vi "read temp.vi"() -> ()   [LabVIEW 2016]
uses:
  <vilib>/Instr/_visa.llb/VISA Configure Serial Port (Instr).vi
panel:
  out "Temperature":dbl[][](graph)
  out "Heater Power":dbl[](graph)
  out "Heater Power":string
  in  "Heater Range":u16(ring) items=["Off", "Low", "Med", "High"]
  in  "Target Temperature":i32
  out "?":string
  out "bytes read":u32
  in  "Set Temperature and heater range":bool
  out "Actual Temperature":string
  in  "Stop Programme":bool
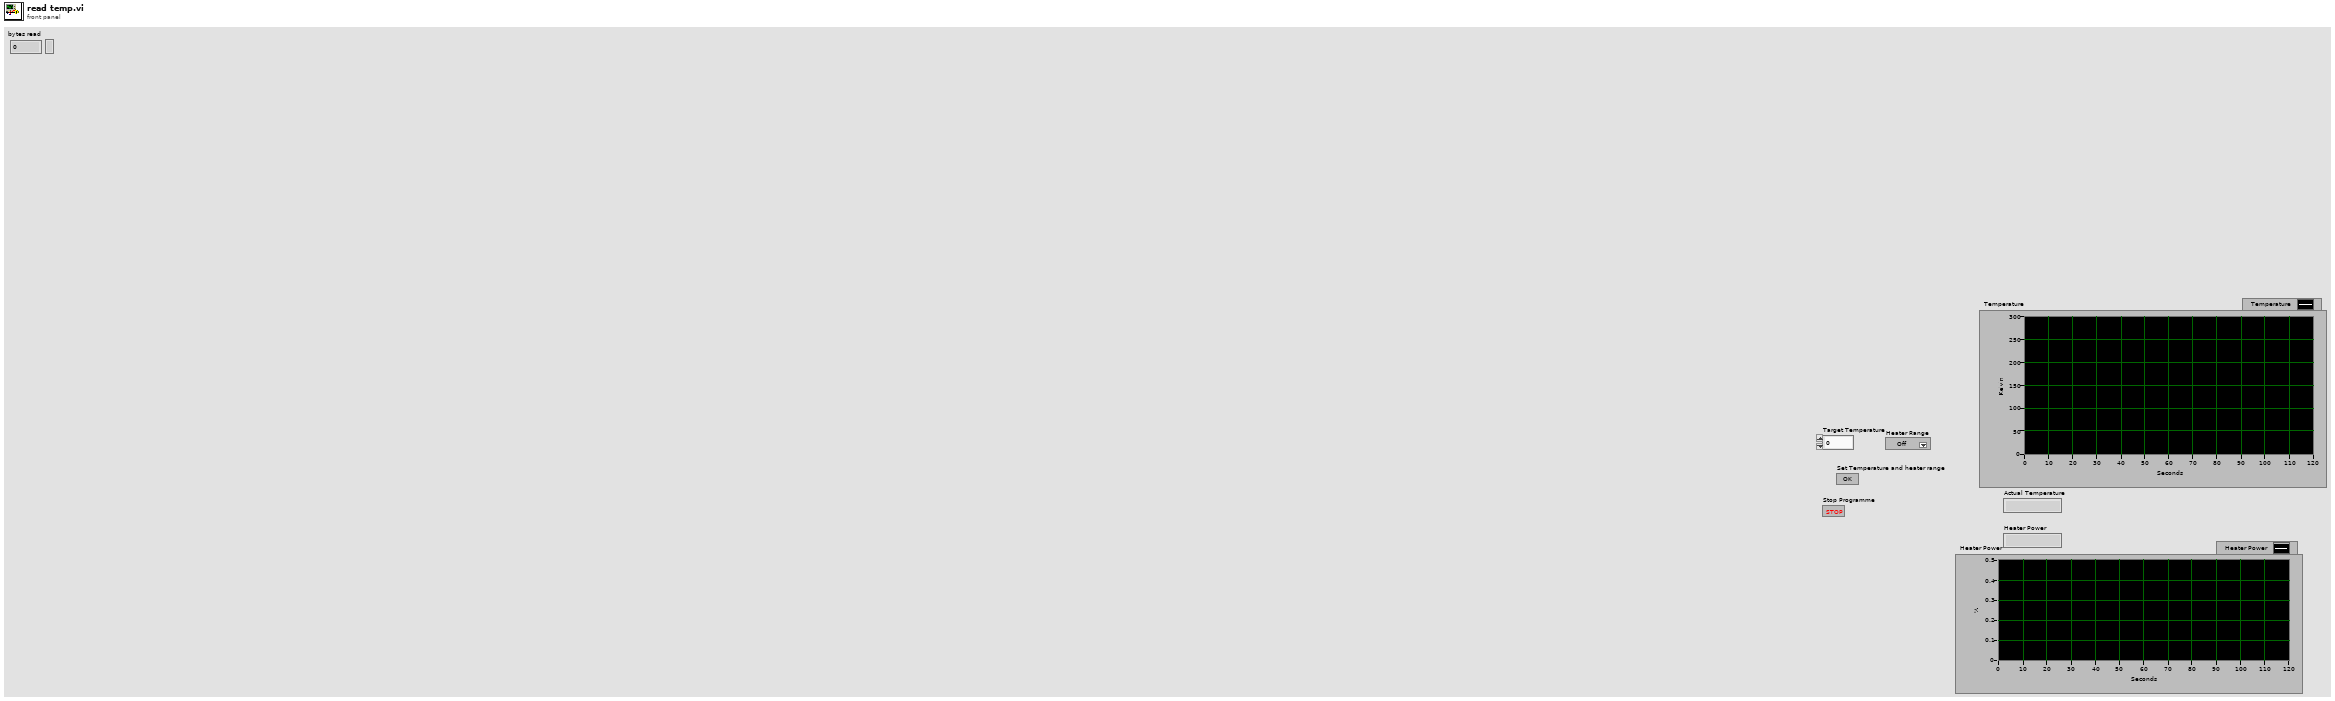
[diagram p1: front panel]
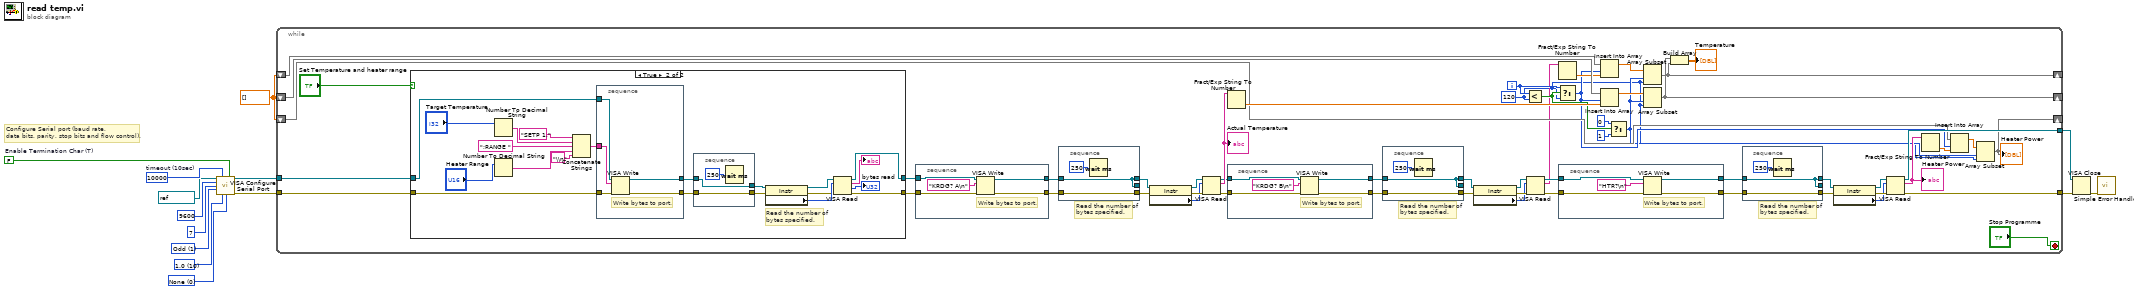
[diagram p0: block diagram]
diagram:
  w1 = dbl[] []
  w7 = u16 0 items=["None"=0, "XON/XOFF"=1, "RTS/CTS"=2, "DTR/DSR"=4] ("flow control")
  w8 = u16 10 items=["1.0"=10, "1.5"=15, "2.0"=20] ("stop bits")
  w9 = u16 1 items=["None", "Odd", "Even", "Mark", "Space"] ("parity")
  w13 = FALSE  # Enable Termination Char (T)
  w14 = u32 10000  # timeout (10sec)
  # "Configure Serial port (baud rate,\ndata bits, parity, stop bits and flow control)."
  n1 = call-poly "VISA Configure Serial Port"("VISA resource name"=refnum<visa-resource-name> "COM3", "timeout (10sec)"=w14, "Enable Termination\nChar (T)"=w13, "baud rate (9600)"=u32 9600 ("baud rate"), "data bits (8)"=u16 7 ("data bits"), "parity (0:none)"=w9, "stop bits (10: 1 bit)"=w8, "flow control (0:none)"=w7) -> ("VISA resource name out"=w5:refnum<visa-resource-name>, "error out"=w4:errorcluster)  [unwired: 1 in, 5 out]
  n2 = while {
    tunnel: w5 -> [w61]
    tunnel: w4 -> [w60]
    tunnel: [w42] -> w3
    tunnel: [w41] -> w2
    shift-right: [w17] -> _
    shift-left: w1 -> [w55]
    shift-right: [w37] -> _
    shift-left: w1 -> [w36]
    shift-right: [w16] -> _
    shift-left: w1 -> [w15]
    i -> [w53]
    stop <- "Stop Programme" stop-if-true
    w19 = 120 ("length")
    # "Read the number of bytes specified."
    # "Read the number of bytes specified."
    # "Read the number of bytes specified."
    n3 = case shown="True" "Set Temperature and heater range" {
      tunnel: w61 -> [w88 w96]
      tunnel: w60 -> [w87 w95]
      tunnel: [w88 w93] -> w59
      tunnel: [w87 w92] -> w58
      frame False {
      }
      frame True {
        # "Read the number of bytes specified."
        n4 = Number To Decimal String(number="Target Temperature") -> (decimal integer string=w109:string)  [unwired: 1 out]
        n5 = Number To Decimal String(number="Heater Range") -> (decimal integer string=w89:string)  [unwired: 1 in]
        n6 = Concatenate Strings("SETP 1,", w109, ";RANGE ", w89, "\\n" ("string")) -> (w99:string)
        n7 = stacked-sequence {
          tunnel: [w117] -> w101
          tunnel: w96 -> [w116]
          tunnel: w95 -> [w115]
          tunnel: [w114] -> w100
          tunnel: w99 -> [w113]
          frame #0 {
            # "Write bytes to port."
            n8 = VISA Write(VISA resource name=w116, write buffer=w113, error in (no error)=w115) -> (VISA resource name out=w114:refnum<visa-resource-name>, error out=w117:errorcluster)  [unwired: 1 out]
          }
        }
        n9 = stacked-sequence {
          tunnel: w101 -> [w112]
          tunnel: [w112] -> w103
          tunnel: w100 -> [w111]
          tunnel: [w111] -> w102
          frame #0 {
            n10 = Wait (ms)(milliseconds to wait=u32 250 ("delay before read (ms)")) -> ()  [unwired: 1 out]
          }
        }
        n11 = property class="Instr"(reference=w102, error in=w103) -> (reference out=w104:refnum<visa-resource-name>, error out=w105:errorcluster, "Serial Settings:Number of Bytes at Serial Port"=w106:u32)
        n12 = VISA Read(VISA resource name=w104, byte count=w106, error in (no error)=w105) -> (VISA resource name out=w93:refnum<visa-resource-name>, read buffer=→"?":string, return count=→"bytes read":u32, error out=w92:errorcluster)
      }
    }
    n13 = stacked-sequence {
      tunnel: [w122] -> w65
      tunnel: [w121] -> w66
      tunnel: w59 -> [w119]
      tunnel: w58 -> [w118]
      frame #0 {
        # "Write bytes to port."
        n14 = VISA Write(VISA resource name=w119, write buffer="KRDG? A\n", error in (no error)=w118) -> (VISA resource name out=w121:refnum<visa-resource-name>, error out=w122:errorcluster)  [unwired: 1 out]
      }
    }
    n15 = stacked-sequence {
      tunnel: w65 -> [w123]
      tunnel: w66 -> [w124]
      tunnel: [w124] -> _
      tunnel: [w124] -> w64
      tunnel: [w123] -> w63
      frame #0 {
        n16 = Wait (ms)(milliseconds to wait=u32 250 ("delay before read (ms) 2")) -> ()  [unwired: 1 out]
      }
    }
    n17 = property class="Instr"(reference=w64, error in=w63) -> (reference out=w70:refnum<visa-resource-name>, error out=w69:errorcluster, "Serial Settings:Number of Bytes at Serial Port"=w68:u32)
    n18 = VISA Read(VISA resource name=w70, byte count=w68, error in (no error)=w69) -> (VISA resource name out=w28:refnum<visa-resource-name>, read buffer=w57:string, error out=w27:errorcluster)  [unwired: 1 out]
    "Actual Temperature" <- w57
    n19 = Fract/Exp String To Number(string=w57) -> (number=w56:dbl)  [unwired: 3 in, 1 out]
    n20 = stacked-sequence {
      tunnel: [w75] -> w31
      tunnel: [w74] -> w32
      tunnel: w28 -> [w72]
      tunnel: w27 -> [w71]
      frame #0 {
        # "Write bytes to port."
        n21 = VISA Write(VISA resource name=w72, write buffer="KRDG? B\n", error in (no error)=w71) -> (VISA resource name out=w74:refnum<visa-resource-name>, error out=w75:errorcluster)  [unwired: 1 out]
      }
    }
    n22 = stacked-sequence {
      tunnel: w31 -> [w76]
      tunnel: w32 -> [w77]
      tunnel: [w77] -> _
      tunnel: [w77] -> w30
      tunnel: [w76] -> w29
      frame #0 {
        n23 = Wait (ms)(milliseconds to wait=u32 250 ("delay before read (ms) 2")) -> ()  [unwired: 1 out]
      }
    }
    n24 = property class="Instr"(reference=w30, error in=w29) -> (reference out=w35:refnum<visa-resource-name>, error out=w34:errorcluster, "Serial Settings:Number of Bytes at Serial Port"=w33:u32)
    n25 = Less?(x=w53, y=w19) -> (x < y?=w50:bool)
    n26 = VISA Read(VISA resource name=w35, byte count=w33, error in (no error)=w34) -> (VISA resource name out=w26:refnum<visa-resource-name>, read buffer=w24:string, error out=w25:errorcluster)  [unwired: 1 out]
    n27 = Fract/Exp String To Number(string=w24) -> (number=w23:dbl)  [unwired: 3 in, 1 out]
    n28 = Select(t=w53, s=w50, f=w19) -> (s? t:f=w22:i32)
    n29 = stacked-sequence {
      tunnel: [w83] -> w45
      tunnel: [w82] -> w46
      tunnel: w26 -> [w80]
      tunnel: w25 -> [w79]
      frame #0 {
        # "Write bytes to port."
        n30 = VISA Write(VISA resource name=w80, write buffer="HTR?\n", error in (no error)=w79) -> (VISA resource name out=w82:refnum<visa-resource-name>, error out=w83:errorcluster)  [unwired: 1 out]
      }
    }
    n31 = Insert Into Array(array=w15, index=w22, new element=w23) -> (w21:dbl[])
    n32 = Insert Into Array(array=w55, index=w22, new element=w56) -> (w54:dbl[])
    n33 = Select(t=0, s=w50, f=1 ("index")) -> (s? t:f=w20:i32)
    n34 = Array Subset(array=w21, index=w20, length=w19) -> (w16:dbl[])
    n35 = Array Subset(array=w54, index=w20, length=w19) -> (w17:dbl[])
    n36 = Build Array(w17, w16) -> (→"Temperature":dbl[][])
    n37 = stacked-sequence {
      tunnel: w45 -> [w84]
      tunnel: w46 -> [w85]
      tunnel: [w85] -> _
      tunnel: [w85] -> w44
      tunnel: [w84] -> w43
      frame #0 {
        n38 = Wait (ms)(milliseconds to wait=u32 250 ("delay before read (ms) 2")) -> ()  [unwired: 1 out]
      }
    }
    n39 = property class="Instr"(reference=w44, error in=w43) -> (reference out=w49:refnum<visa-resource-name>, error out=w48:errorcluster, "Serial Settings:Number of Bytes at Serial Port"=w47:u32)
    n40 = VISA Read(VISA resource name=w49, byte count=w47, error in (no error)=w48) -> (VISA resource name out=w42:refnum<visa-resource-name>, read buffer=w38:string, error out=w41:errorcluster)  [unwired: 1 out]
    "Heater Power" <- w38
    n41 = Fract/Exp String To Number(string=w38) -> (number=w40:dbl)  [unwired: 3 in, 1 out]
    n42 = Insert Into Array(array=w36, index=w22, new element=w40) -> (w39:dbl[])
    n43 = Array Subset(array=w39, index=w20, length=w19) -> (w37:dbl[])
    "Heater Power" <- w37
  }
  n44 = VISA Close(VISA resource name=w3, error in (no error)=w2) -> (error out=w6:errorcluster)
  n45 = call <vilib>:"Simple Error Handler.vi"("error in (no error)"=w6) -> ()  [unwired: 1 in, 8 out]
